vi "Play with Global1play.vi"() -> ()   [LabVIEW 2014]
uses:
  Global1play.vi
panel:
  in  "stop":bool
  in  "n1":dbl
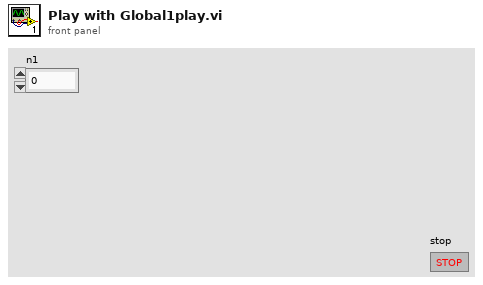
[diagram p1: front panel]
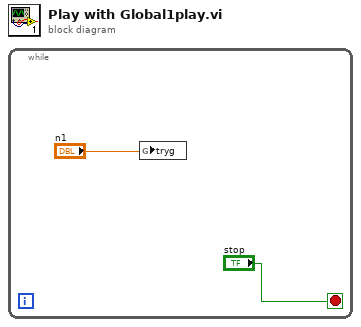
[diagram p0: block diagram]
diagram:
  n1 = while {
    stop <- "stop" stop-if-true
    n2 = global write "Global1play.vi" "tryg"("n1") -> ()
  }
